vi "PPR_Begin.vi"(8 "error in":errorcluster) -> (0 "error out":errorcluster)   [LabVIEW 2019]
doc: "Called before other user functions, this VI is expected to open initial I/O refnums, load in file data, and do all program initialization. Notice that the <B>error out</B> terminal is simply used for data flow. Wiring it to other structures or subVIs ensures that this VI runs first."
uses:
  PPR_Robot Global Data.vi
  <vilib>/Rock Robotics/WPI/DriverStation/WPI_DriverStationRobotMode2.ctl
  <vilib>/Rock Robotics/Network Tables/NT Write String Array.vi
  <vilib>/Rock Robotics/WPI/ThirdParty/JAS_Junk/TrajLib/Trajectory_Library.lvlib
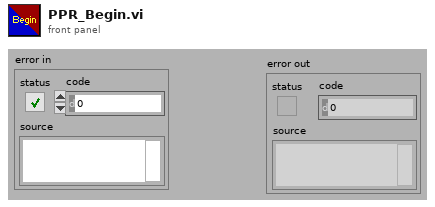
[diagram p1: front panel]
types:
  T1 = typedef "WPI_DriverStationRobotMode2.ctl" = enum16{"Autonomous Disabled", "Autonomous Enabled", "Teleop Disabled", "Teleop Enabled", "Disconnected", "Finish", "Test Disabled", "Test Enabled", "Emergency Stopped"}
  T2 = typedef "Trajectory_Library.lvlib/ROTATION2D.ctl" = cluster{"VALUE":dbl, "COS":dbl, "SIN":dbl}
  T3 = typedef "Trajectory_Library.lvlib/POSE2D.ctl" = cluster{"TRANSLATION":T4, "ROTATION":T2}
  T4 = typedef "Trajectory_Library.lvlib/TRANSLATION2D.ctl" = cluster{"X":dbl, "Y":dbl}
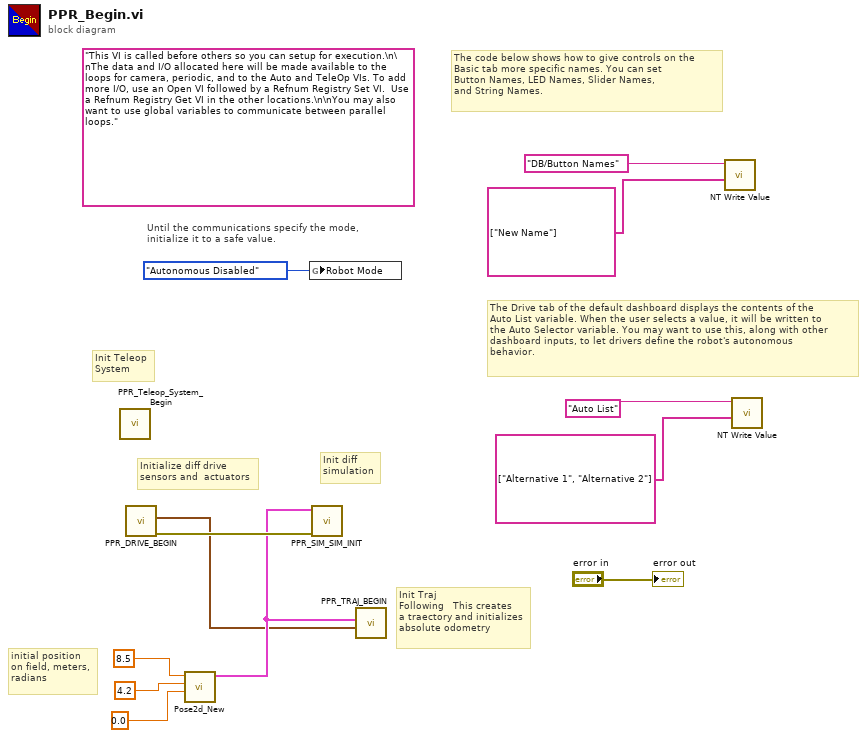
[diagram p0: block diagram]
diagram:
  (unwired) "This VI is called before others so you can setup for execution.\n\nThe data and I/O allocated here will be made available to the loops for camera, periodic, and to the Auto and TeleOp VIs. To add more I/O, use an Open VI followed by a Refnum Registry Set VI.  Use a Refnum Registry Get VI in the other locations.\n\nYou may also want to use global variables to communicate between parallel loops."
  # "Init diff\nsimulation"
  # "Init Teleop \nSystem"
  # "Init Traj\nFollowing   This creates\na traectory and initializes\nabsolute odometry"
  # "Initialize diff drive\nsensors and  actuators"
  # "initial position\non field, meters,\nradians"
  # "The Drive tab of the default dashboard displays the contents of the\nAuto List variable. When the user selects a value, it will be written to\nthe Auto Selector variable. You may want to use this, along with other\ndashboard inputs, to let drivers define the robot's autonomous\nbehavior."
  # "The code below shows how to give controls on the\nBasic tab more specific names. You can set\nButton Names, LED Names, Slider Names,\nand String Names."
  # "Until the communications specify the mode,\ninitialize it to a safe value."
  n1 = call "PPR_Teleop_System_Begin.vi"() -> ()  [unwired: 12 in]
  n2 = call "PPR_DRIVE_BEGIN.vi"() -> ("error out"=w3:errorcluster, "Gyro Reading"=w1:T2)  [unwired: 9 in, 1 out]
  n3 = call <vilib>:"Pose2d_New.vi"("Heading"=0.0, "Y"=4.2, "X"=8.5) -> ("out POSe"=w2:T3)  [unwired: 8 in]
  n4 = global write "PPR_Robot Global Data.vi" "Robot Mode"(WPI_DriverStationRobotMode2."Autonomous Disabled" ("Robot Mode")) -> ()
  n5 = call "PPR_SIM_SIM_INIT.vi"("error in (no error)"=w3, "Initial Robot Position"=w2) -> ()  [unwired: 9 in, 1 out]
  n6 = call "PPR_TRAJ_BEGIN.vi"("Initial Gyo Reading"=w1, "Robot Starting Pose"=w2) -> ()  [unwired: 10 in]
  n7 = call-poly <vilib>:"NT Write Value.vi"("value"=string[] ["New Name"], "name"="DB/Button Names" ("Name")) -> ()  [unwired: 9 in, 1 out]
  n8 = call-poly <vilib>:"NT Write Value.vi"("value"=string[] ["Alternative 1", "Alternative 2"] ("String Array"), "name"="Auto List" ("Name")) -> ()  [unwired: 9 in, 1 out]
  "error out" <- "error in"
